vi "WPI_AccelerometerADXL362_SPI_Get.vi"(8 "error in":errorcluster, 11 "AccelerometerDevRef":T2={"DevStatus"={"status"=FALSE, "code"=0, "source"=""}, "Scaling"={"Gain (VoltsPerG)"=0.0, "Center Voltage"=0.0}, "Analog Channels"={"X-Axis"=enum."Invalid", "Y-Axis"=enum."Invalid", "Z-Axis"=enum."Invalid"}, "I2C Bus"=enum."Invalid", "SPI Bus"=enum."Invalid", "Accel Range"=0, "ADXL Axes"={"X-Axis"=FALSE, "Y-Axis"=FALSE, "Z-Axis"=FALSE}, "Handle"=0, "Device Address"=0, "Accel Type"=enum."Analog"} {"Device Address" format="%.0x"; "Accel Range" items=["+/- 2 g", "+/- 4 g", "+/- 8 g", "+/- 16 g"]}) -> (0 "error out":errorcluster, 2 "Accelerations":T1, 3 "AccelerometerDevRef":T2={"DevStatus"={"status"=FALSE, "code"=0, "source"=""}, "Scaling"={"Gain (VoltsPerG)"=0.0, "Center Voltage"=0.0}, "Analog Channels"={"X-Axis"=enum."Invalid", "Y-Axis"=enum."Invalid", "Z-Axis"=enum."Invalid"}, "I2C Bus"=enum."Invalid", "SPI Bus"=enum."Invalid", "Accel Range"=0, "ADXL Axes"={"X-Axis"=FALSE, "Y-Axis"=FALSE, "Z-Axis"=FALSE}, "Handle"=0, "Device Address"=0, "Accel Type"=enum."Analog"} {"Device Address" format="%.0x"; "Accel Range" items=["+/- 2 g", "+/- 4 g", "+/- 8 g", "+/- 16 g"]})   [LabVIEW 2017]
doc: "Returns the current acceleration of the sensor that you specify.\n\nThis software is licensed. Open the labview\\readme\\WPI Robotics Library Open Source License.txt file for more information."
uses:
  <vilib>/Rock Robotics/WPI/Accelerometer/WPI_AccelerometerDevRef.ctl
  <vilib>/Rock Robotics/WPI/Accelerometer/WPI_AccelerometerScaling.ctl
  <vilib>/Rock Robotics/WPI/Accelerometer/WPI_AccelerometerAnalogChannels.ctl
  <vilib>/Rock Robotics/SystemInterfaces/AI/FPGA_AIChannel.ctl
  <vilib>/Rock Robotics/SystemInterfaces/i2clib/i2c_bus.ctl
  <vilib>/Rock Robotics/SystemInterfaces/spilib/spi_bus.ctl
  <vilib>/Rock Robotics/WPI/Accelerometer/ADXL345 Range.ctl
  <vilib>/Rock Robotics/WPI/Accelerometer/WPI_AccelerometerADXL345 Axes.ctl
  <vilib>/Rock Robotics/WPI/SPI/WPI_SPIDevRef.ctl
panel:
  # "ADXL"
  # "Analog"
  # "ADXL"
  # "Analog"
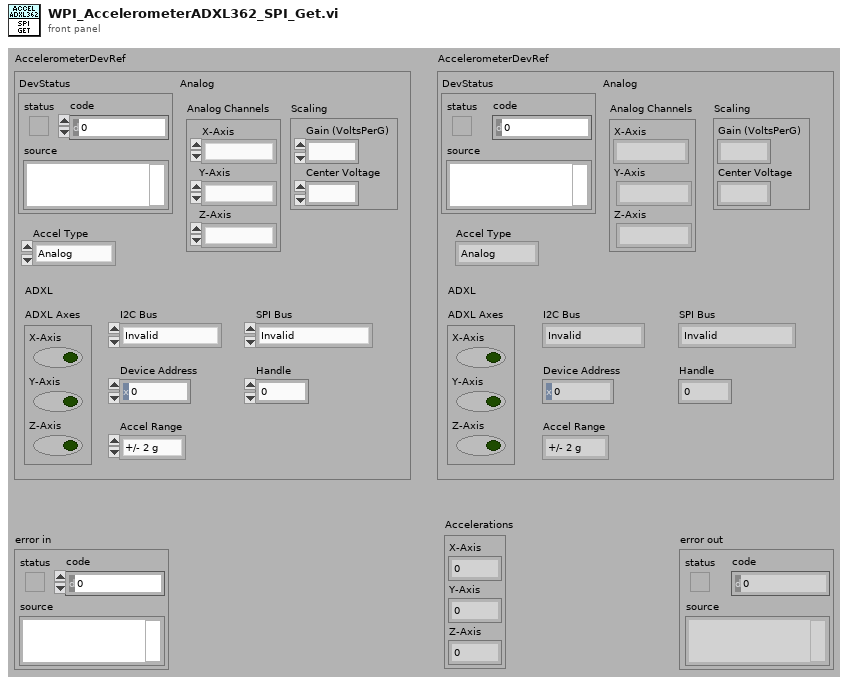
[diagram p1: front panel]
types:
  T1 = cluster{"X-Axis":dbl, "Y-Axis":dbl, "Z-Axis":dbl}
  T2 = typedef "WPI_AccelerometerDevRef.ctl" = cluster{"DevStatus":errorcluster, "Scaling":T3, "Analog Channels":T4, "I2C Bus":T6, "SPI Bus":T7, "Accel Range":T8, "ADXL Axes":T9, "Handle":i32, "Device Address":u8, "Accel Type":enum16{"Analog", "ADXL345 I2C", "ADXL345 SPI", "Internal", "ADXL362 SPI"}}
  T3 = typedef "WPI_AccelerometerScaling.ctl" = cluster{"Gain (VoltsPerG)":dbl, "Center Voltage":dbl}
  T4 = typedef "WPI_AccelerometerAnalogChannels.ctl" = cluster{"X-Axis":T5, "Y-Axis":T5, "Z-Axis":T5}
  T5 = typedef "FPGA_AIChannel.ctl" = enum8{"AI 0", "AI 1", "AI 2", "AI 3", "AI MXP 0", "AI MXP 1", "AI MXP 2", "AI MXP 3", "Invalid"}
  T6 = typedef "i2c_bus.ctl" = enum16{"I2C On-Board", "I2C MXP", "Invalid"}
  T7 = typedef "spi_bus.ctl" = enum16{"SPI On-Board, CS0", "SPI On-Board, CS1", "SPI On-Board, CS2", "SPI On-Board, CS3", "SPI MXP", "Invalid"}
  T8 = typedef "ADXL345 Range.ctl" = u8
  T9 = typedef "WPI_AccelerometerADXL345 Axes.ctl" = cluster{"X-Axis":bool, "Y-Axis":bool, "Z-Axis":bool}
  T10 = typedef "WPI_SPIDevRef.ctl" = cluster{"DevStatus":errorcluster, "Handle":i32, "SPI Bus":T7}
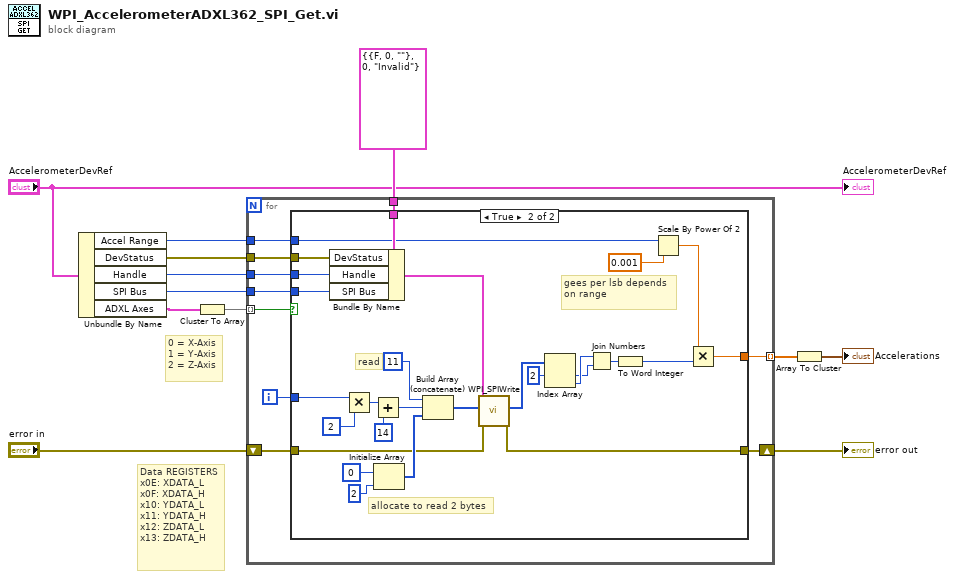
[diagram p0: block diagram]
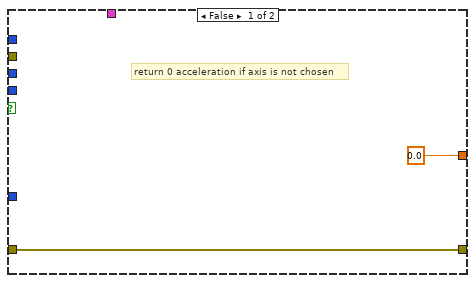
[diagram p2: hidden frame]
diagram:
  # "Data REGISTERS\nx0E: XDATA_L\nx0F: XDATA_H\nx10: YDATA_L\nx11: YDATA_H\nx12: ZDATA_L\nx13: ZDATA_H"
  # "0 = X-Axis\n1 = Y-Axis\n2 = Z-Axis"
  n1 = Unbundle By Name("AccelerometerDevRef") -> ("Accel Range"=w1:T8, "DevStatus"=w9:errorcluster, "Handle"=w10:i32, "SPI Bus"=w7:T7, "ADXL Axes"=w5:T9)
  n2 = Cluster To Array(cluster=w5) -> (array=w4:bool[])
  n3 = for {
    shift-right: [w22] -> w12
    shift-left: "error in" -> [w21]
    tunnel: T10 {"DevStatus"={"status"=FALSE, "code"=0, "source"=""}, "Handle"=0, "SPI Bus"=enum."Invalid"} ("SPIDevRef") -> [w20]
    tunnel: w10 -> [w19]
    tunnel: w9 -> [w18]
    tunnel: w7 -> [w17]
    tunnel: [w16] -> w6 mode=indexing
    tunnel: w4 -> [w15] mode=indexing
    tunnel: w1 -> [w13]
    i -> [w14]
    n4 = case shown="True" w15 {
      tunnel: [w24 w33] -> w22
      tunnel: w21 -> [w24 w34]
      tunnel: w20 -> [_ w51]
      tunnel: w19 -> [_ w50]
      tunnel: w18 -> [_ w49]
      tunnel: w17 -> [_ w48]
      tunnel: [0.0 ("Voltage") w35] -> w16
      tunnel: w14 -> [_ w37]
      tunnel: w13 -> [_ w27]
      frame False {
        # "return 0 acceleration if axis is not chosen"
      }
      frame True {
        # "gees per lsb depends on range"
        # "allocate to read 2 bytes"
        # "read"
        n5 = Bundle By Name(cluster=w51, "DevStatus"=w49, "Handle"=w50, "SPI Bus"=w48) -> (w36:T10)
        n6 = Multiply(x=w37, y=u32 2 ("Data To Send")) -> (x*y=w47:u32)
        n7 = Add(x=w47, y=u32 14 ("Data To Send")) -> (x+y=w30:u32)
        n8 = Initialize Array(u8 0 ("Data To Send"), 2 ("dimension size")) -> (w44:u8[])
        n9 = Build Array (concatenate)(u8 11 ("Data To Send"), w30, w44) -> (w43:u32[])
        n10 = call <vilib>:"WPI_SPIWrite.vi"("error in (no error)"=w34, "Data To Send"=w43, "SPIDevRef"=w36) -> ("error out"=w33:errorcluster, "Received Data"=w42:u8[])  [unwired: 7 out]
        n11 = Index Array(array=w42, index #1=2 ("index")) -> (element #1=w38:u8, element #2=w39:u8)  [unwired: 1 in]
        n12 = Join Numbers(hi=w39, lo=w38) -> ((hi.lo)=w40:u16)
        n13 = To Word Integer(number=w40) -> (16bit integer=w28:i16)
        n14 = Scale By Power Of 2(n=w27, x=0.001 ("y")) -> (x*2^n=w25:dbl)
        n15 = Multiply(x=w25, y=w28) -> (x*y=w35:dbl)
      }
    }
  }
  "error out" <- w12
  n16 = Array To Cluster(array=w6) -> (cluster=→"Accelerations":cluster{"[0]":dbl, "[1]":dbl, "[2]":dbl})
  "AccelerometerDevRef" <- "AccelerometerDevRef"
